vi "AdminLogIn(SubVI).vi"() -> ()   [LabVIEW 2013]
panel:
  in  "Add More Attempts":bool
  in  "Set the No Of Attempts":bool
  in  "Set the Number of Questions":bool
  in  "Show Student's Login/out History":bool
  in  "Go Back":bool
  in  "Administrator no":string
  in  "Administrrator Password":string
  in  "Login":bool
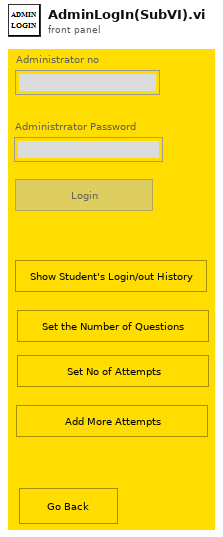
[diagram p1: front panel]
types:
  T1 = enum8{"Enabled", "Disabled", "Disabled and Grayed Out"}
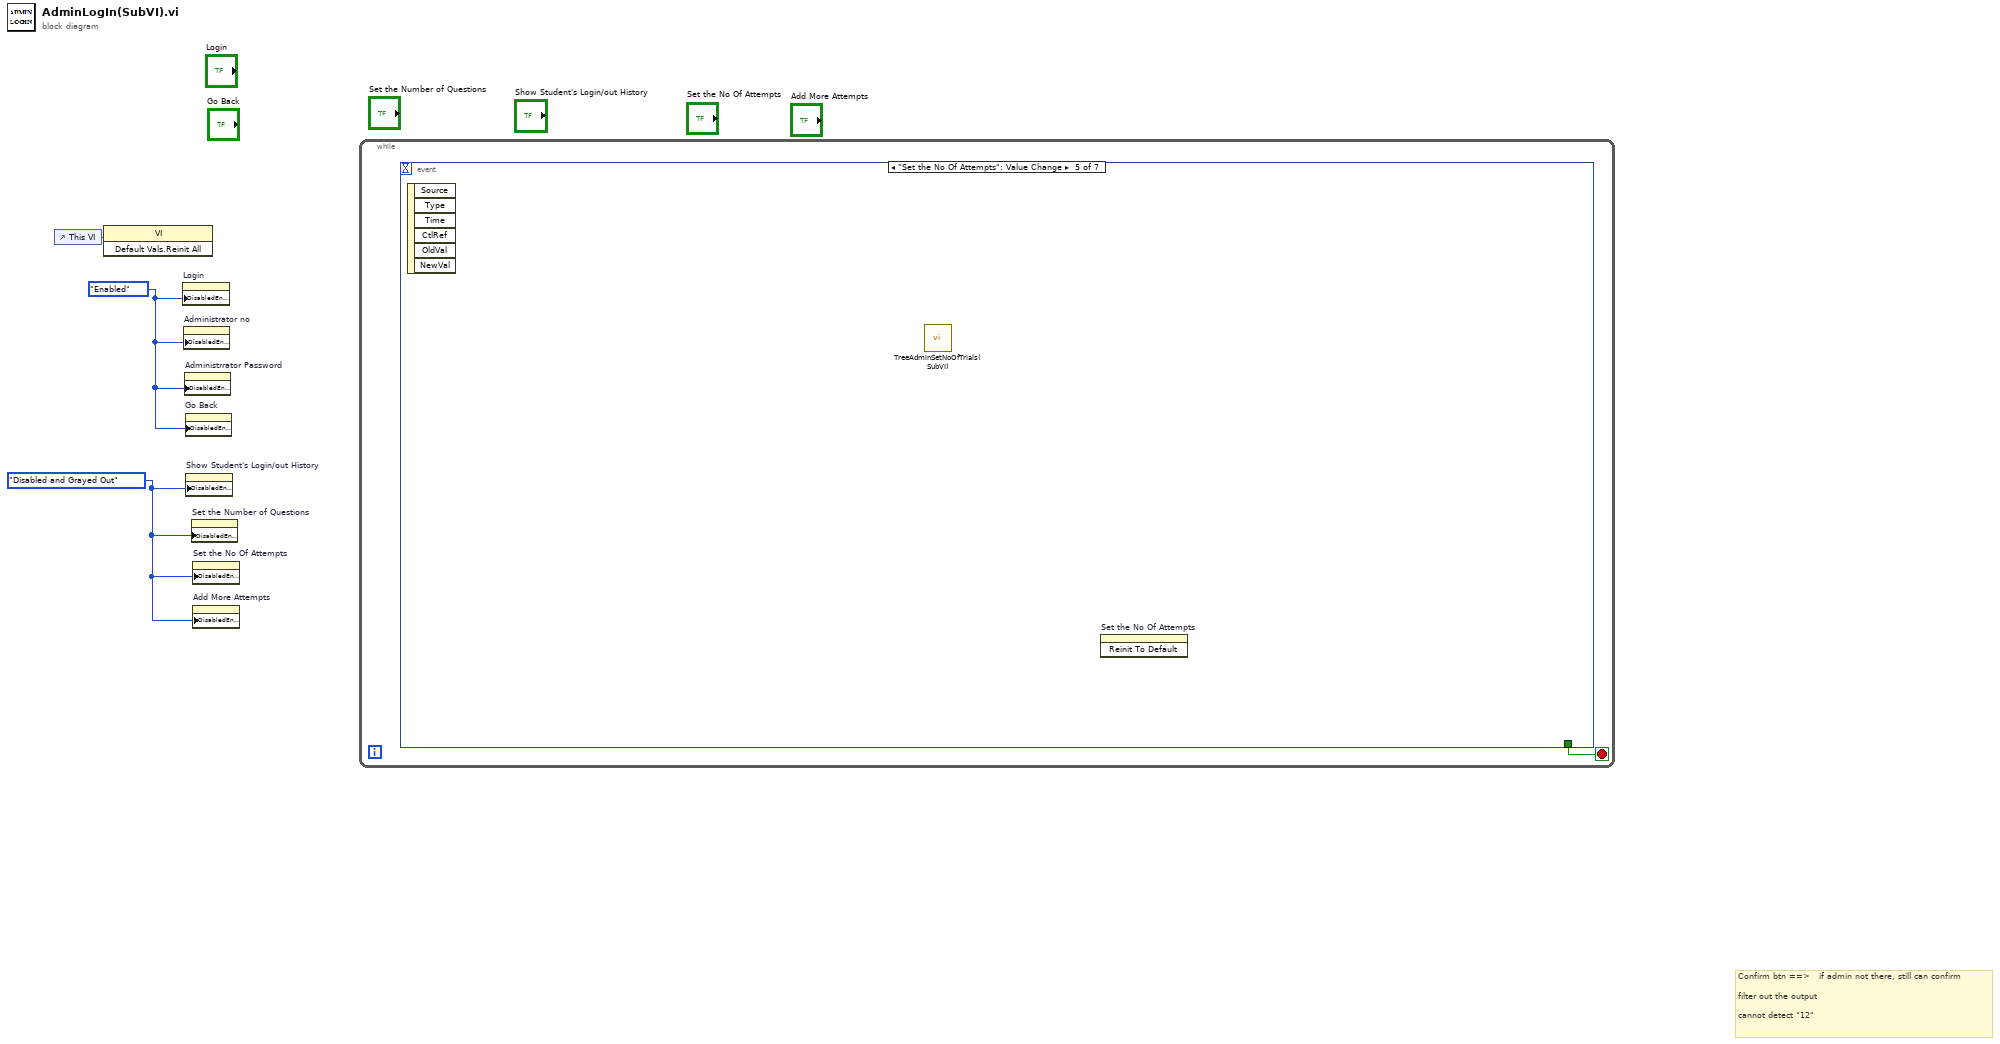
[diagram p0: block diagram]
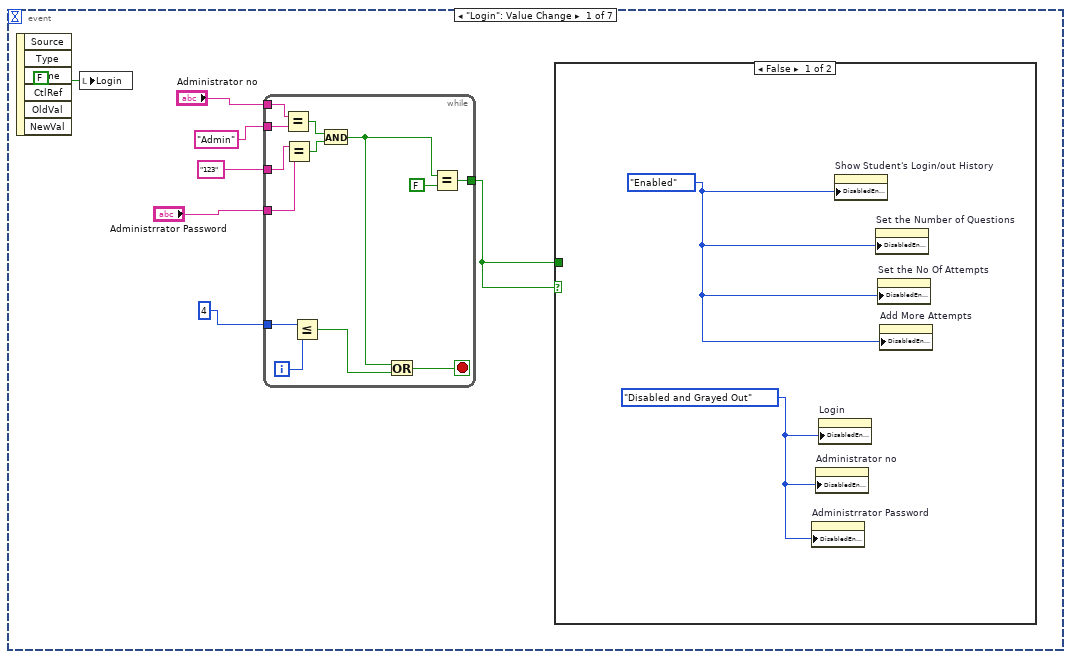
[diagram p2: hidden frame]
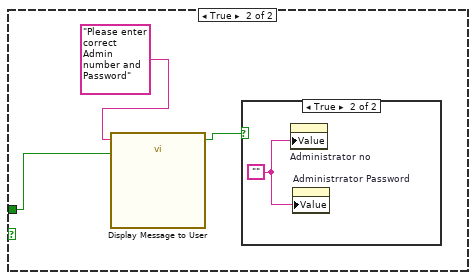
[diagram p3: hidden frame]
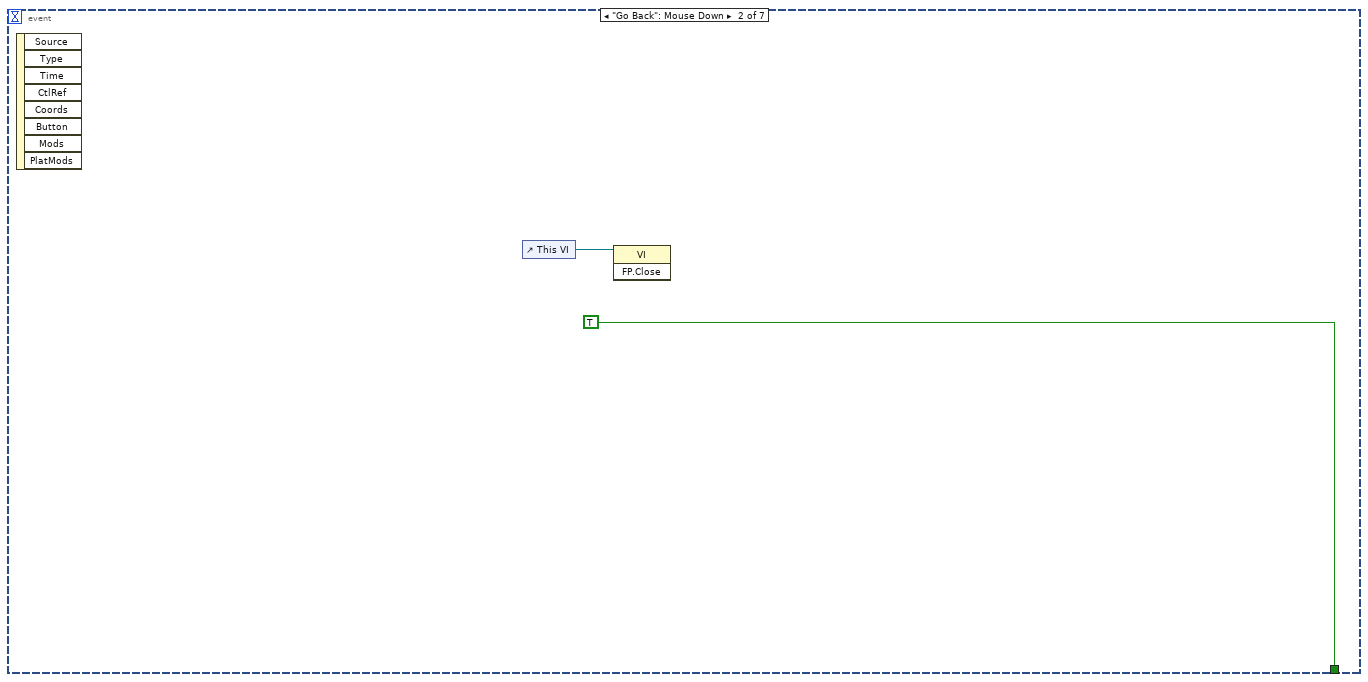
[diagram p5: hidden frame]
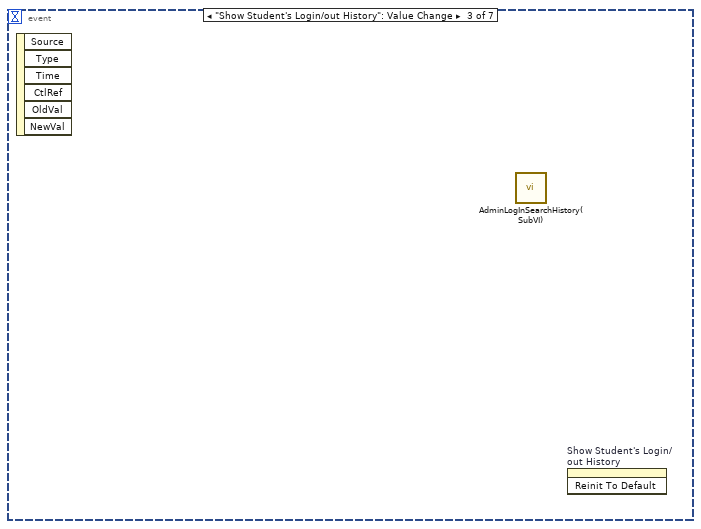
[diagram p6: hidden frame]
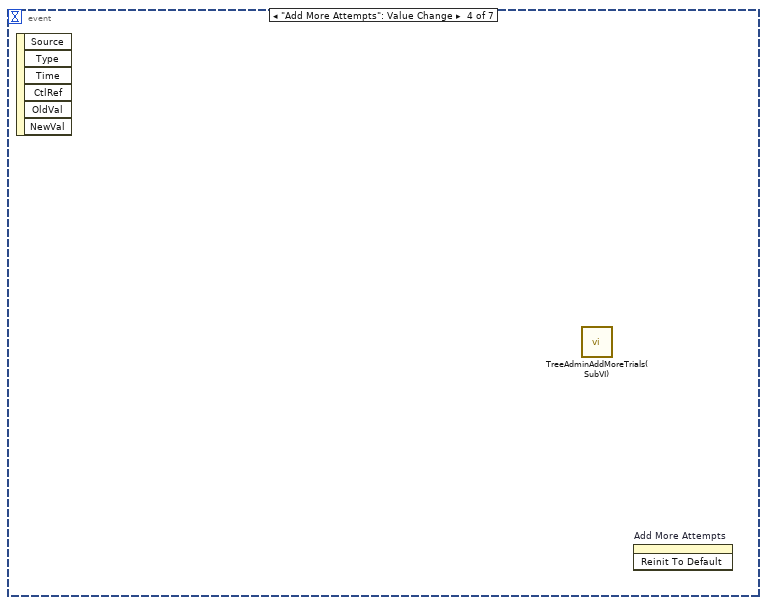
[diagram p7: hidden frame]
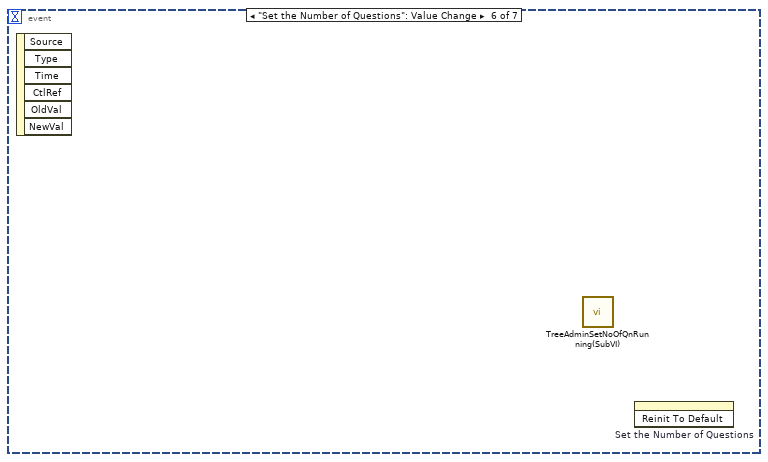
[diagram p8: hidden frame]
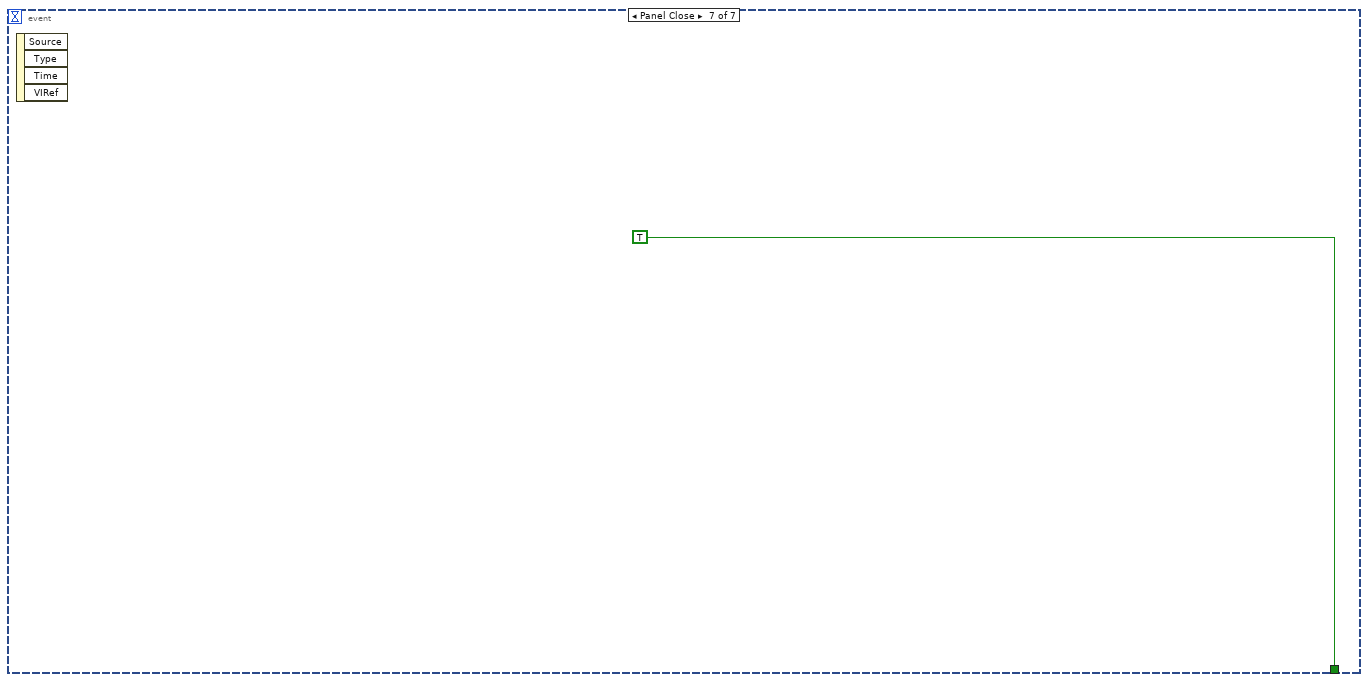
[diagram p9: hidden frame]
diagram:
  w1 = T1."Disabled and Grayed Out"
  w2 = T1."Enabled"
  # "Confirm btn ==>   if admin not there, still can confirm\n\nfilter out the output\n\ncannot detect \"12\""
  n1 = control-ref of="This VI"() -> (w3:refnum<vi>)
  n2 = invoke class="VI" method="Default Vals.Reinit All"(reference=w3) -> ()  [unwired: 2 in, 3 out]
  n3 = property on="Login" class="Bool (strict)"("DisabledEnum"=w2) -> ()  [unwired: 2 in, 2 out]
  n4 = property on="Administrator no" class="Str"("DisabledEnum"=w2) -> ()  [unwired: 2 in, 2 out]
  n5 = property on="Administrrator Password" class="Str"("DisabledEnum"=w2) -> ()  [unwired: 2 in, 2 out]
  n6 = property on="Go Back" class="Bool (strict)"("DisabledEnum"=w2) -> ()  [unwired: 2 in, 2 out]
  n7 = property on="Show Student's Login/out History" class="Bool (strict)"("DisabledEnum"=w1) -> ()  [unwired: 2 in, 2 out]
  n8 = property on="Set the Number of Questions" class="Bool (strict)"("DisabledEnum"=w1) -> ()  [unwired: 2 in, 2 out]
  n9 = property on="Set the No Of Attempts" class="Bool (strict)"("DisabledEnum"=w1) -> ()  [unwired: 2 in, 2 out]
  n10 = property on="Add More Attempts" class="Bool (strict)"("DisabledEnum"=w1) -> ()  [unwired: 2 in, 2 out]
  n11 = while {
    stop <- w4 stop-if-true
    n12 = event shown="[4] \"Set the No Of Attempts\": Value Change" {
      selector: _ -> [_ _ _ _ _ _ _]
      dyn-events: _ -> [_ _ _ _ _ _ _]
      timeout: _ -> [_ _ _ _ _ _ _]
      tunnel: [_ TRUE _ _ _ _ TRUE] -> w4
      event "Login": Value Change {
        n13 = event-data() -> ()  [unwired: 1 in, 6 out]
        n14 = local write "Login"(FALSE) -> ()
        n15 = while {
          tunnel: "Administrator no" -> [w26]
          tunnel: "Administrrator Password" -> [w27]
          tunnel: [w25] -> w5
          tunnel: "Admin" -> [w24]
          tunnel: "123" -> [w23]
          tunnel: 4 -> [w22]
          i -> [w21]
          stop <- w18 stop-if-true
          n16 = Equal?(x=w26, y=w24) -> (x = y?=w30:bool)
          n17 = Equal?(x=w23, y=w27) -> (x = y?=w29:bool)
          n18 = Less Or Equal?(x=w22, y=w21) -> (x <= y?=w19:bool)
          n19 = And(x=w30, y=w29) -> (x .and. y?=w20:bool)
          n20 = Or(x=w20, y=w19) -> (x .or. y?=w18:bool)
          n21 = Equal?(x=w20, y=FALSE) -> (x = y?=w25:bool)
        }
        n22 = case shown="False" w5 {
          tunnel: w5 -> [_ w15]
          frame False {
            w13 = T1."Disabled and Grayed Out"
            w12 = T1."Enabled"
            n23 = property on="Administrrator Password" class="Str"("DisabledEnum"=w13) -> ()  [unwired: 2 in, 2 out]
            n24 = property on="Administrator no" class="Str"("DisabledEnum"=w13) -> ()  [unwired: 2 in, 2 out]
            n25 = property on="Login" class="Bool (strict)"("DisabledEnum"=w13) -> ()  [unwired: 2 in, 2 out]
            n26 = property on="Show Student's Login/out History" class="Bool (strict)"("DisabledEnum"=w12) -> ()  [unwired: 2 in, 2 out]
            n27 = property on="Set the Number of Questions" class="Bool (strict)"("DisabledEnum"=w12) -> ()  [unwired: 2 in, 2 out]
            n28 = property on="Set the No Of Attempts" class="Bool (strict)"("DisabledEnum"=w12) -> ()  [unwired: 2 in, 2 out]
            n29 = property on="Add More Attempts" class="Bool (strict)"("DisabledEnum"=w12) -> ()  [unwired: 2 in, 2 out]
          }
          frame True {
            n30 = call "Display Message to User"("Enable"=w15, "Message"="Please enter correct Admin number and Password") -> ("OK"=w14:bool)  [unwired: 8 in, 1 out]
            n31 = case shown="True" w14 {
              frame False {
              }
              frame True {
                w17 = ""
                n32 = property on="Administrator no" class="Str"("Value"=w17) -> ()  [unwired: 2 in, 2 out]
                n33 = property on="Administrrator Password" class="Str"("Value"=w17) -> ()  [unwired: 2 in, 2 out]
              }
            }
          }
        }
      }
      event "Go Back": Mouse Down {
        n34 = event-data() -> ()  [unwired: 1 in, 8 out]
        n35 = control-ref of="This VI"() -> (w32:refnum<vi>)
        n36 = invoke class="VI" method="FP.Close"(reference=w32) -> ()  [unwired: 2 in, 3 out]
      }
      event "Show Student's Login/out History": Value Change {
        n37 = event-data() -> ()  [unwired: 1 in, 6 out]
        n38 = call "AdminLogInSearchHistory(SubVI).vi"() -> ()  [unwired: 12 in]
        n39 = invoke on="Show Student's Login/out History" class="Bool (strict)" method="Reinit To Default"() -> ()  [unwired: 3 in, 3 out]
      }
      event "Add More Attempts": Value Change {
        n40 = event-data() -> ()  [unwired: 1 in, 6 out]
        n41 = call "TreeAdminAddMoreTrials(SubVI).vi"() -> ()  [unwired: 12 in]
        n42 = invoke on="Add More Attempts" class="Bool (strict)" method="Reinit To Default"() -> ()  [unwired: 3 in, 3 out]
      }
      event "Set the No Of Attempts": Value Change {
        n43 = event-data() -> ()  [unwired: 1 in, 6 out]
        n44 = call "TreeAdminSetNoOfTrials(SubVI).vi"() -> ()  [unwired: 12 in]
        n45 = invoke on="Set the No Of Attempts" class="Bool (strict)" method="Reinit To Default"() -> ()  [unwired: 3 in, 3 out]
      }
      event "Set the Number of Questions": Value Change {
        n46 = event-data() -> ()  [unwired: 1 in, 6 out]
        n47 = call "TreeAdminSetNoOfQnRunning(SubVI).vi"() -> ()  [unwired: 12 in]
        n48 = invoke on="Set the Number of Questions" class="Bool (strict)" method="Reinit To Default"() -> ()  [unwired: 3 in, 3 out]
      }
      event Panel Close {
        n49 = event-data() -> ()  [unwired: 1 in, 4 out]
      }
    }
  }
